vi "Reset_db_for_new_waveforms.vi"() -> ()   [LabVIEW 2013]
panel:
  out "Query String":string
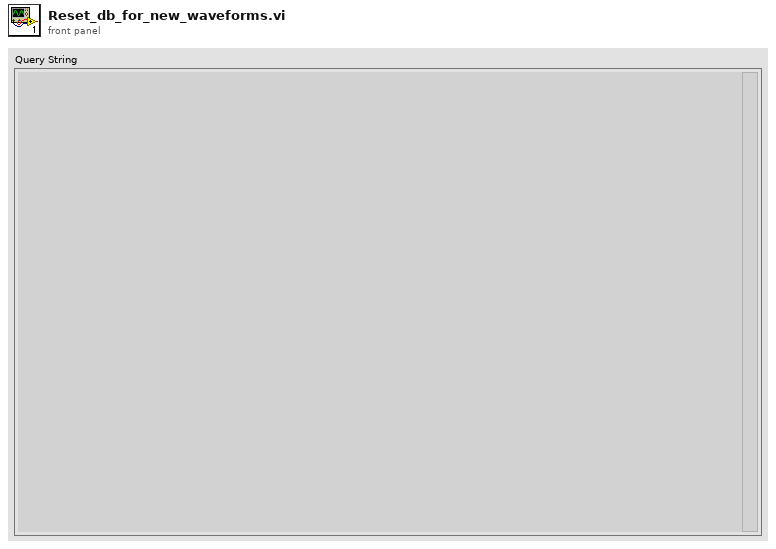
[diagram p1: front panel]
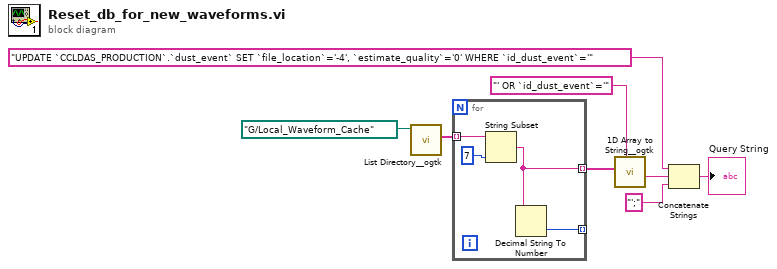
[diagram p0: block diagram]
diagram:
  n1 = call <userlib>:"List Directory__ogtk.vi"("directory path"=path "G:/Local_Waveform_Cache") -> ("file names"=w8:string[])  [unwired: 3 in, 3 out]
  n2 = for {
    tunnel: w8 -> [w12] mode=indexing
    tunnel: [w10] -> w6 mode=indexing
    tunnel: [w9] -> _ mode=indexing
    n3 = String Subset(string=w12, length (rest)=7 ("length (rest)")) -> (substring=w10:string)  [unwired: 1 in]
    n4 = Decimal String To Number(string=w10) -> (number=w9:i32)  [unwired: 2 in, 1 out]
  }
  n5 = call <userlib>:"1D Array to String__ogtk.vi"("delimiter (Tab)"="' OR `id_dust_event`='", "Array of Strings"=w6) -> ("delimited string"=w4:string)  [unwired: 9 in]
  n6 = Concatenate Strings("UPDATE `CCLDAS_PRODUCTION`.`dust_event` SET `file_location`='-4', `estimate_quality`='0' WHERE `id_dust_event`='" ("string"), w4, "';" ("string")) -> (→"Query String":string)
